vi "CMD_Will.vi"(8 "error in (no error)":errorcluster, 9 "IP":string="172.16.0.248", 10 "MAC":string="0050C500001E", 11 "HOSTNAME":string="SI-AGT01") -> (0 "error out":errorcluster, 3 "UpdatedJSON":string)   [LabVIEW 2020]
uses:
  <vilib>/addons/JSON API/JSON Value/Set from JSON string.vi
  <vilib>/LabVIEW Open Source Project/Epoch Date & Time/epoch.UNIX/Epoch.UNIX.lvclass
  C:/Program Files/National Instruments/LabVIEW 2020/vi.lib/LabVIEW Open Source Project/Epoch Date & Time/epoch/Epoch.lvclass
  <vilib>/addons/JSON API/JSON Scalar/JSON Scalar.lvclass
  C:/Program Files/National Instruments/LabVIEW 2020/vi.lib/addons/JSON API/JSON Value/JSON Value.lvclass
  <vilib>/addons/JSON API/JSON Array/JSON Array.lvclass
  <vilib>/LabVIEW Open Source Project/Epoch Date & Time/Get Epoch Time.vi
  <vilib>/addons/JSON API/JSON Scalar/Set I64.vi
  <vilib>/addons/JSON API/JSON Scalar/Set String.vi
  <vilib>/addons/JSON API/JSON Value/Get Array by name.vi
  <vilib>/addons/JSON API/JSON Array/Set JSON Array.vi
  <vilib>/addons/JSON API/JSON Value/JSON Value.lvclass
  <vilib>/addons/JSON API/Get Polymorphic/JSON GetSet.lvlib
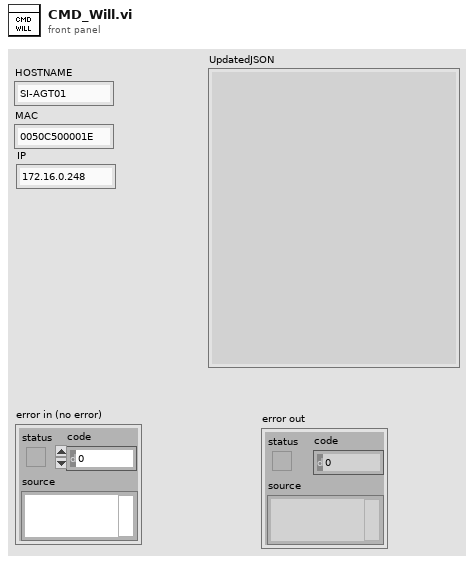
[diagram p1: front panel]
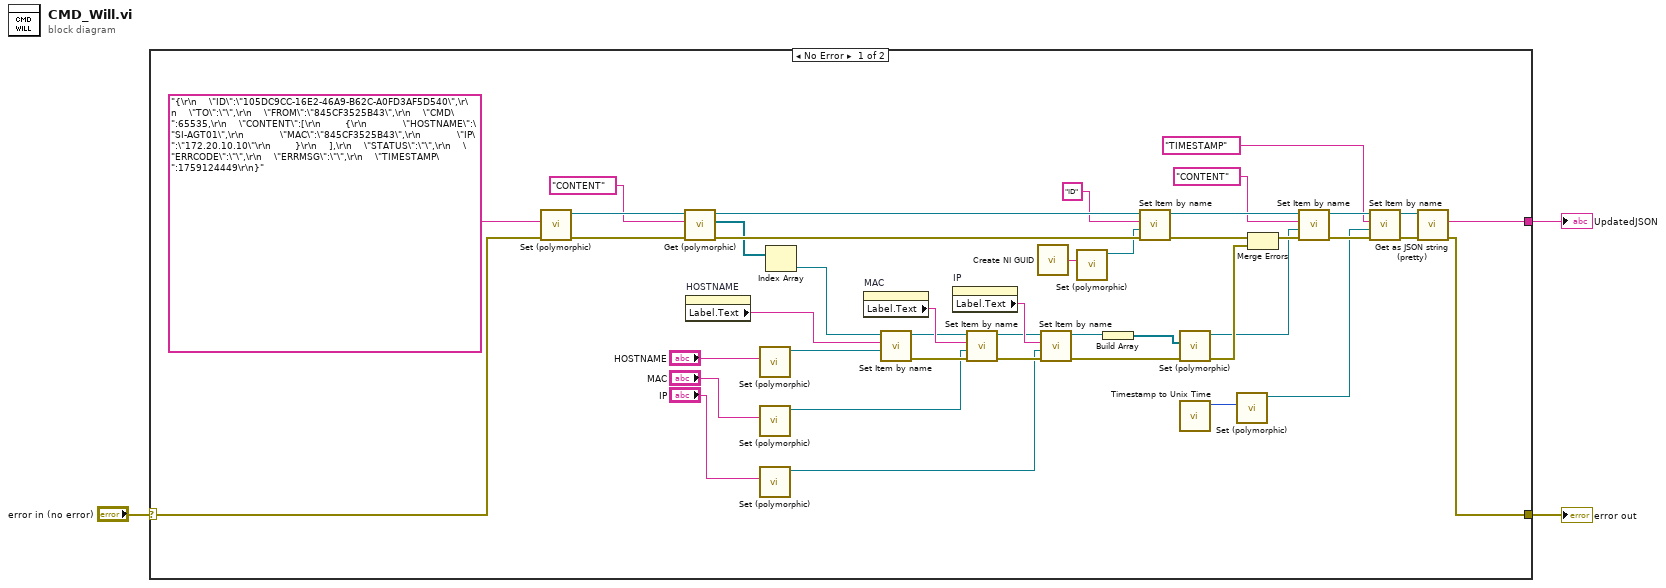
[diagram p0: block diagram]
diagram:
  n1 = case shown="No Error" "error in (no error)" {
    selector: "error in (no error)" -> [w4 w47]
    tunnel: [w5 w47] -> w3
    tunnel: [w6 _] -> w1
    frame No Error {
      n2 = call-poly <vilib>:"Set (polymorphic).vi"("error in (no error)"=w4, "JSON stream"="{\r\n    \"ID\":\"105DC9CC-16E2-46A9-B62C-A0FD3AF5D540\",\r\n    \"TO\":\"\",\r\n    \"FROM\":\"845CF3525B43\",\r\n    \"CMD\":65535,\r\n    \"CONTENT\":[\r\n        {\r\n            \"HOSTNAME\":\"SI-AGT01\",\r\n            \"MAC\":\"845CF3525B43\",\r\n            \"IP\":\"172.20.10.10\"\r\n        }\r\n    ],\r\n    \"STATUS\":\"\",\r\n    \"ERRCODE\":\"\",\r\n    \"ERRMSG\":\"\",\r\n    \"TIMESTAMP\":1759124449\r\n}" ("JSON String")) -> ("error out"=w37:errorcluster, "JSON Value out"=w29:refnum<class "JSON Value.lvclass">)  [unwired: 7 in, 1 out]
      n3 = call-poly <vilib>:"Get (polymorphic).vi"("error in (no error)"=w37, "name"="CONTENT", "JSON Value In"=w29) -> ("error out"=w38:errorcluster, "Array"=w30:refnum<class "JSON Value.lvclass">[], "JSON Value Out"=w36:refnum<class "JSON Value.lvclass">)  [unwired: 5 in, 1 out]
      n4 = property on="HOSTNAME" class="Str"() -> ("Label.Text"=w22:string)  [unwired: 2 in, 2 out]
      n5 = call-poly <vilib>:"Set (polymorphic).vi"("String"="HOSTNAME") -> ("JSON Scalar out"=w19:refnum<class "JSON Scalar.lvclass">)  [unwired: 9 in, 1 out]
      n6 = call-poly <vilib>:"Set (polymorphic).vi"("String"="MAC") -> ("JSON Scalar out"=w24:refnum<class "JSON Scalar.lvclass">)  [unwired: 9 in, 1 out]
      n7 = call-poly <vilib>:"Set (polymorphic).vi"("String"="IP") -> ("JSON Scalar out"=w26:refnum<class "JSON Scalar.lvclass">)  [unwired: 9 in, 1 out]
      n8 = Index Array(array=w30) -> (element=w31:refnum<class "JSON Value.lvclass">)  [unwired: 1 in]
      n9 = property on="MAC" class="Str"() -> ("Label.Text"=w23:string)  [unwired: 2 in, 2 out]
      n10 = call-dynamic "Set Item by name.vi"("Value"=w19, "name"=w22, "JSON Value In"=w31) -> ("error out"=w42:errorcluster, "JSON Value Out"=w20:refnum<class "JSON Value.lvclass">)  [unwired: 6 in, 1 out]
      n11 = property on="IP" class="Str"() -> ("Label.Text"=w25:string)  [unwired: 2 in, 2 out]
      n12 = call-dynamic "Set Item by name.vi"("error in (no error)"=w42, "Value"=w24, "name"=w23, "JSON Value In"=w20) -> ("error out"=w43:errorcluster, "JSON Value Out"=w21:refnum<class "JSON Value.lvclass">)  [unwired: 5 in, 1 out]
      n13 = call <vilib>:"Create NI GUID.vi"() -> ("NI GUID"=w12:string)
      n14 = call-dynamic "Set Item by name.vi"("error in (no error)"=w43, "Value"=w26, "name"=w25, "JSON Value In"=w21) -> ("error out"=w44:errorcluster, "JSON Value Out"=w27:refnum<class "JSON Value.lvclass">)  [unwired: 5 in, 1 out]
      n15 = call-poly <vilib>:"Set (polymorphic).vi"("String"=w12) -> ("JSON Scalar out"=w13:refnum<class "JSON Scalar.lvclass">)  [unwired: 9 in, 1 out]
      n16 = Build Array(w27) -> (w28:refnum<class "JSON Value.lvclass">[])
      n17 = call-dynamic "Set Item by name.vi"("error in (no error)"=w38, "Value"=w13, "name"="ID", "JSON Value In"=w36) -> ("error out"=w39:errorcluster, "JSON Value Out"=w14:refnum<class "JSON Value.lvclass">)  [unwired: 5 in, 1 out]
      n18 = call-poly <vilib>:"Set (polymorphic).vi"("error in (no error)"=w44, "Array"=w28) -> ("error out"=w46:errorcluster, "JSON Array out"=w15:refnum<class "JSON Array.lvclass">)  [unwired: 8 in]
      n19 = call <vilib>:"Timestamp to Unix Time.vi"() -> ("Unix Time (s)"=w34:i64)  [unwired: 10 in, 1 out]
      n20 = call-poly <vilib>:"Set (polymorphic).vi"("Numeric"=w34) -> ("JSON Scalar out"=w35:refnum<class "JSON Scalar.lvclass">)  [unwired: 9 in, 1 out]
      n21 = Merge Errors(w39, w46) -> (w45:errorcluster)
      n22 = call-dynamic "Set Item by name.vi"("error in (no error)"=w45, "Value"=w15, "name"="CONTENT", "JSON Value In"=w14) -> ("error out"=w40:errorcluster, "JSON Value Out"=w32:refnum<class "JSON Value.lvclass">)  [unwired: 5 in, 1 out]
      n23 = call-dynamic "Set Item by name.vi"("error in (no error)"=w40, "Value"=w35, "name"="TIMESTAMP", "JSON Value In"=w32) -> ("error out"=w41:errorcluster, "JSON Value Out"=w33:refnum<class "JSON Value.lvclass">)  [unwired: 5 in, 1 out]
      n24 = call <vilib>:"Get as JSON string (pretty).vi"("error in (no error)"=w41, "JSON Value in"=w33) -> ("error out"=w5:errorcluster, "<JSON>"=w6:string)  [unwired: 8 in]
    }
    frame Error {
    }
  }
  "error out" <- w3
  "UpdatedJSON" <- w1
